vi "Update_colunter_bottles.vi"(6 "Available data names":string[](array[string]), 11 "Odour bottles in":T1(array[cluster])) -> (3 "Odour bottles out":T1(array[cluster]))   [LabVIEW 2016]
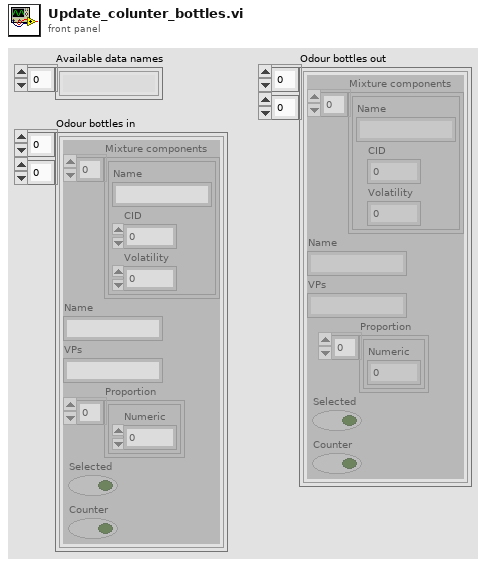
[diagram p1: front panel]
types:
  T1 = cluster{"Mixture components":cluster{"Name":string, "CID":i32, "Volatility":dbl}[], "Name":string, "VPs":string, "Proportion":cluster{"Numeric":dbl}[], "Selected":bool, "Counter":bool}[][]
  T2 = cluster{"Mixture components":cluster{"Name":string, "CID":i32, "Volatility":dbl}[], "Name":string, "VPs":string, "Proportion":cluster{"Numeric":dbl}[], "Selected":bool, "Counter":bool}
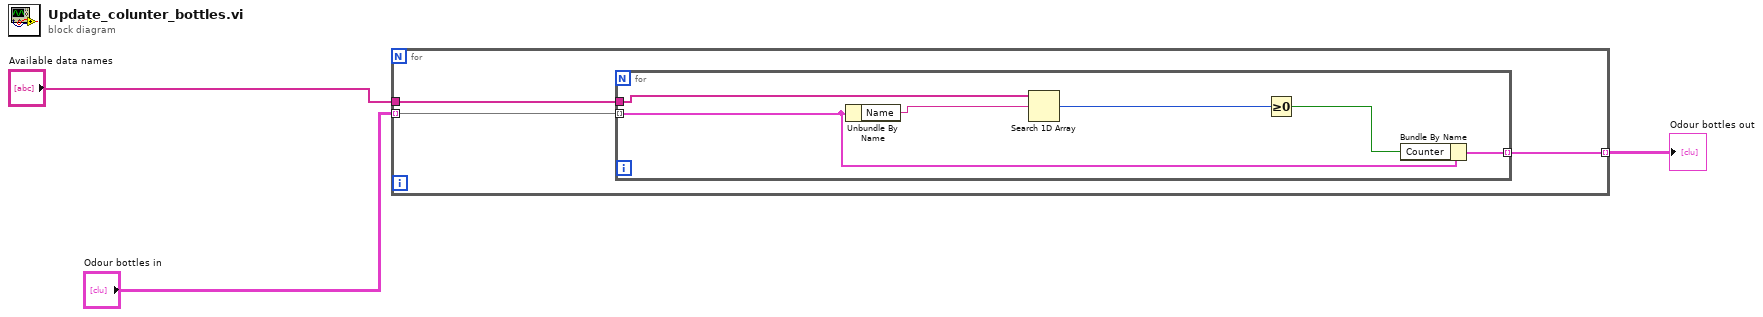
[diagram p0: block diagram]
diagram:
  n1 = for {
    tunnel: "Odour bottles in" -> [w6] mode=indexing
    tunnel: [w5] -> w2 mode=indexing
    tunnel: "Available data names" -> [w4]
    n2 = for {
      tunnel: w6 -> [w12] mode=indexing
      tunnel: [w7] -> w5 mode=indexing
      tunnel: w4 -> [w10]
      n3 = Unbundle By Name(w12) -> ("Name"=w11:string)
      n4 = Search 1D Array(1D array=w10, element=w11) -> (index of element=w9:i32)  [unwired: 1 in]
      n5 = Greater Or Equal To 0?(x=w9) -> (x >= 0?=w8:bool)
      n6 = Bundle By Name(cluster=w12, "Counter"=w8) -> (w7:T2)
    }
  }
  "Odour bottles out" <- w2
